vi "配置信息迁移.vi"(8 "error in (no error)":errorcluster) -> (0 "error out":errorcluster)   [LabVIEW 2022 SP3, in "斯坦道总氮V2.lvlib"]
uses:
  <vilib>/Utility/config.llb/Read Key (String).vi
  <vilib>/Utility/config.llb/Write Key (String).vi
  <vilib>/Utility/config.llb/NI_LVConfig.lvlib
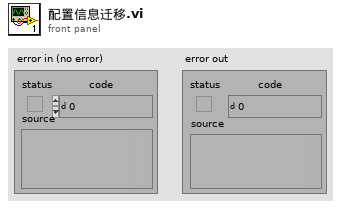
[diagram p1: front panel]
types:
  T1 = typedef "NI_LVConfig.lvlib/Config Data RefNum.ctl" = refnum<k1>
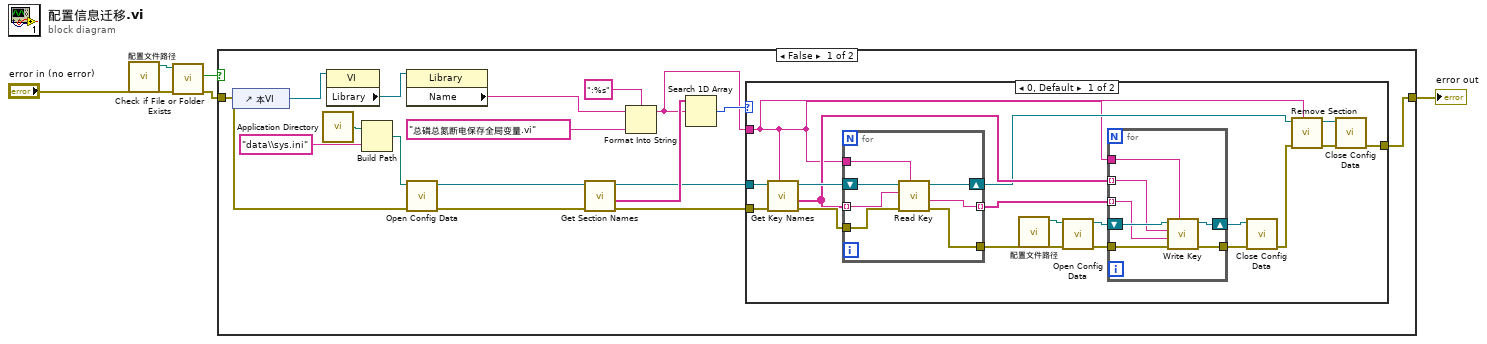
[diagram p0: block diagram]
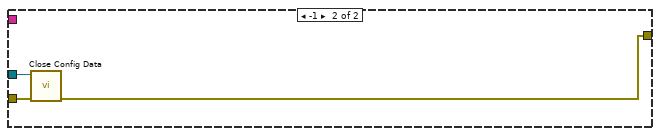
[diagram p2: hidden frame]
diagram:
  n1 = call "配置文件路径.vi"() -> ("appended path"=w5:path)  [unwired: 11 in]
  n2 = call <vilib>:"Check if File or Folder Exists.vi"("error in (no error)"="error in (no error)", "path"=w5) -> ("error out"=w2:errorcluster, "file or folder exists?"=w4:bool)  [unwired: 7 in, 1 out]
  n3 = case shown="False" w4 {
    tunnel: w2 -> [w7 w58]
    tunnel: [w6 w58] -> w1
    frame False {
      n4 = control-ref of="本VI"() -> (w18:refnum<vi>)
      n5 = call <vilib>:"Application Directory.vi"() -> ("Application Directory"=w20:path)
      n6 = property class="VI"(reference=w18) -> ("Library"=w17:refnum<vi>)  [unwired: 1 in, 2 out]
      n7 = Build Path(base path=w20, name or relative path="data\\sys.ini" ("名称或相对路径")) -> (appended path=w19:path)
      n8 = property class="Library"(reference=w17) -> ("Name"=w16:string)  [unwired: 1 in, 2 out]
      n9 = call <vilib>:"Open Config Data.vi"("error in (no error)"=w7, "configuration file path"=w19) -> ("error out"=w12:errorcluster, "refnum"=w22:T1)  [unwired: 7 in, 1 out]
      n10 = call <vilib>:"Get Section Names.vi"("error in (no error)"=w12, "refnum"=w22) -> ("error out"=w10:errorcluster, "section names"=w13:string[], "refnum out"=w11:T1)  [unwired: 7 in]
      n11 = Format Into String(format string=":%s" ("格式字符串"), initial string=w16, "总磷总氮断电保存全局变量.vi" ("section (optional)")) -> (resulting string=w8:string)  [unwired: 1 in, 1 out]
      n12 = Search 1D Array(1D array=w13, element=w8) -> (index of element=w9:i32)  [unwired: 1 in]
      n13 = case shown="0, Default" w9 {
        tunnel: w11 -> [w40 w57]
        tunnel: w10 -> [w39 w56]
        tunnel: w8 -> [w25 _]
        tunnel: [w23 w55] -> w6
        frame 0, Default {
          n14 = call <vilib>:"Get Key Names.vi"("section"=w25, "error in (no error)"=w39, "refnum"=w40) -> ("error out"=w37:errorcluster, "key names"=w36:string[], "refnum out"=w38:T1)  [unwired: 5 in, 1 out]
          n15 = for {
            tunnel: w37 -> [w53]
            tunnel: w36 -> [w52] mode=indexing
            tunnel: w25 -> [w51]
            shift-right: [w50] -> w28
            shift-left: w38 -> [w54]
            tunnel: [w49] -> w27
            tunnel: [w48] -> w35 mode=indexing
            n16 = call-poly <vilib>:"Read Key.vi"("section"=w51, "error in (no error)"=w53, "key"=w52, "refnum"=w54) -> ("error out"=w49:errorcluster, "value"=w48:string, "refnum out"=w50:T1)  [unwired: 4 in, 1 out]
          }
          n17 = call "配置文件路径.vi"() -> ("appended path"=w30:path)  [unwired: 11 in]
          n18 = call <vilib>:"Open Config Data.vi"("error in (no error)"=w27, "configuration file path"=w30) -> ("error out"=w33:errorcluster, "refnum"=w34:T1)  [unwired: 7 in, 1 out]
          n19 = for {
            tunnel: w36 -> [w41] mode=indexing
            tunnel: w35 -> [w46] mode=indexing
            tunnel: w25 -> [w45]
            tunnel: w33 -> [w44]
            shift-right: [w43] -> w32
            shift-left: w34 -> [w47]
            tunnel: [w42] -> w31
            n20 = call-poly <vilib>:"Write Key.vi"("section"=w45, "error in (no error)"=w44, "value"=w46, "key"=w41, "refnum"=w47) -> ("error out"=w42:errorcluster, "refnum out"=w43:T1)  [unwired: 4 in, 1 out]
          }
          n21 = call <vilib>:"Close Config Data.vi"("error in (no error)"=w31, "refnum"=w32) -> ("error out"=w29:errorcluster)  [unwired: 8 in, 1 out]
          n22 = call <vilib>:"Remove Section.vi"("section"=w25, "error in (no error)"=w29, "refnum"=w28) -> ("error out"=w26:errorcluster, "refnum out"=w24:T1)  [unwired: 6 in, 1 out]
          n23 = call <vilib>:"Close Config Data.vi"("error in (no error)"=w26, "refnum"=w24) -> ("error out"=w23:errorcluster)  [unwired: 8 in, 1 out]
        }
        frame -1 {
          n24 = call <vilib>:"Close Config Data.vi"("error in (no error)"=w56, "refnum"=w57) -> ("error out"=w55:errorcluster)  [unwired: 8 in, 1 out]
        }
      }
    }
    frame True {
    }
  }
  "error out" <- w1
